vi "Add Text.vi"(8 "Error In":errorcluster, 11 "Parser In":refnum<class "Parser.lvclass">) -> (0 "Error Out":errorcluster, 3 "Parser Out":refnum<class "Parser.lvclass">)   [LabVIEW 2017, in "Mustache.lvlib" / "Parser.lvclass"]
uses:
  Parser.lvclass
  Parser.lvclass/Parser.ctl
  Public/Controls/Token.ctl
  Public/Controls/Token Types.ctl
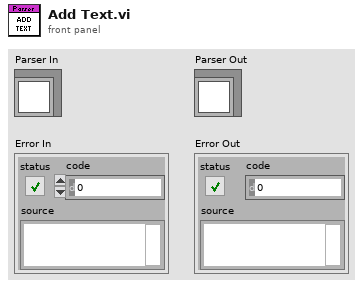
[diagram p1: front panel]
types:
  T1 = typedef "Mustache.lvlib/Parser.lvclass/Token.ctl" = cluster{"Type":T2, "Data":variant}
  T2 = typedef "Mustache.lvlib/Parser.lvclass/Token Types.ctl" = enum16{"Text", "Escaped Tag", "Unescaped Tag", "Section", "Incomplete Section", "Partial"}
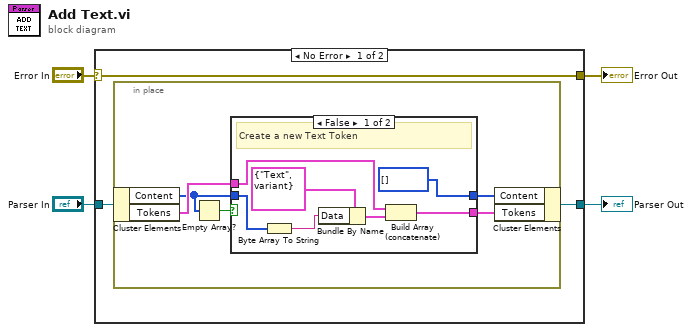
[diagram p0: block diagram]
diagram:
  n1 = case shown="No Error" "Error In" {
    selector: "Error In" -> [w5 w22]
    tunnel: "Parser In" -> [w7 w23]
    tunnel: [w6 w23] -> w1
    tunnel: [w5 w22] -> w2
    frame No Error {
      n2 = in-place {
        n3 = in-place-cluster #1(w7) -> ("Content"=w10:u8[], "Tokens"=w11:T1[])
        n4 = Empty Array?(array=w10) -> (empty?=w12:bool)
        n5 = case shown="False" w12 {
          tunnel: w10 -> [w18 w20]
          tunnel: w11 -> [w16 w21]
          tunnel: [w14 w21] -> w8
          tunnel: [u8[] [] ("Content") w20] -> w9
          frame False {
            # "Create a new Text Token"
            n6 = Byte Array To String(unsigned byte array=w18) -> (string=w17:string)
            n7 = Bundle By Name(cluster=T1 {"Type"=enum."Text", "Data"=variant} ("Token"), "Data"=w17) -> (w15:T1)
            n8 = Build Array (concatenate)(w16, w15) -> (w14:T1[])
          }
          frame True {
            # "The content is part of the tag, not text"
          }
        }
        n9 = in-place-cluster #1("Content"=w9, "Tokens"=w8) -> (w6:refnum<class "Parser.lvclass">)
      }
    }
    frame Error {
    }
  }
  "Error Out" <- w2
  "Parser Out" <- w1
